vi "DriverStationSim_Comm_Loop.vi"(8 "error in (no error)":errorcluster) -> ()   [LabVIEW 2019, in "Trajectory_Library.lvlib"]
uses:
  Trajectory_Library.lvlib
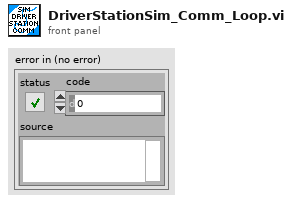
[diagram p1: front panel]
types:
  T1 = typedef "WPI_DriverStationRobotMode2.ctl" = enum16{"Autonomous Disabled", "Autonomous Enabled", "Teleop Disabled", "Teleop Enabled", "Disconnected", "Finish", "Test Disabled", "Test Enabled", "Emergency Stopped"}
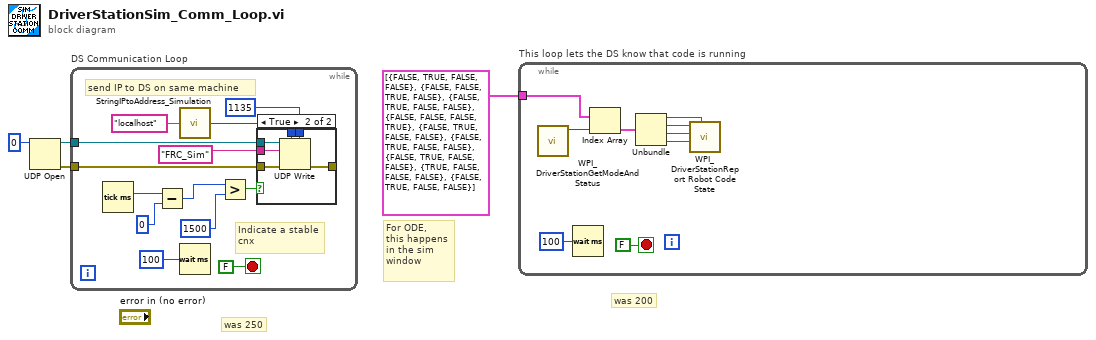
[diagram p0: block diagram]
diagram:
  # "was 200"
  # "was 250"
  # "For ODE,\nthis happens\nin the sim\nwindow"
  n1 = UDP Open(11:u16 0 ("port")) -> (port=w4:refnum<k16>, 0:w3:errorcluster)  [unwired: 4 in, 1 out]
  n2 = while "DS Communication Loop" {
    tunnel: w4 -> [w16]
    tunnel: w3 -> [w17]
    stop <- FALSE stop-if-true
    # "Indicate a stable\ncnx"
    # "send IP to DS on same machine"
    n3 = Tick Count (ms)() -> (millisecond timer value=w6:u32)
    n4 = Subtract(x=w6, y=u32 0) -> (x-y=w9:u32)
    n5 = call <vilib>:"StringIPtoAddress_Simulation.vi"("string IP"="localhost" ("DS IP 2")) -> ("address"=w13:u32)  [unwired: 14 in]
    n6 = Wait (ms)(milliseconds to wait=u32 100) -> ()  [unwired: 1 out]
    n7 = Greater?(x=w9, y=u32 1500 ("milliseconds to wait")) -> (0:w7:bool)
    n8 = case shown="True" w7 {
      tunnel: w17 -> [_ w23]
      tunnel: w16 -> [_ w22]
      tunnel: "FRC_Sim" ("data in") -> [_ w21]
      tunnel: w13 -> [_ w20]
      tunnel: [_ w19] -> _
      tunnel: u16 1135 ("port") -> [_ w18]
      frame False {
      }
      frame True {
        n9 = UDP Write(address=w20, port or service name=w18, connection ID=w22, data in=w21, 8:w23) -> (error out=w19:errorcluster)  [unwired: 1 in, 1 out]
      }
    }
  }
  n10 = while "This loop lets the DS know that code is running" {
    tunnel: cluster{bool, bool, bool, bool}[] [{FALSE, TRUE, FALSE, FALSE}, {FALSE, FALSE, TRUE, FALSE}, {FALSE, TRUE, FALSE, FALSE}, {FALSE, FALSE, FALSE, TRUE}, {FALSE, TRUE, FALSE, FALSE}, {FALSE, TRUE, FALSE, FALSE}, {FALSE, TRUE, FALSE, FALSE}, {TRUE, FALSE, FALSE, FALSE}, {FALSE, TRUE, FALSE, FALSE}] -> [w31]
    stop <- FALSE stop-if-true
    n11 = call <vilib>:"WPI_DriverStationGetModeAndStatus.vi"() -> ("Robot Mode"=w25:T1)  [unwired: 10 in, 1 out]
    n12 = Wait (ms)(milliseconds to wait=u32 100) -> ()  [unwired: 1 out]
    n13 = Index Array(array=w31, index=w25) -> (element=w26:cluster{bool, bool, bool, bool})
    n14 = Unbundle(w26) -> (w32:bool, w24:bool, w29:bool, w28:bool)
    n15 = call <vilib>:"WPI_DriverStationReport Robot Code State.vi"("Test"=w32, "TeleOp"=w28, "Autonomous"=w29, "Disabled"=w24) -> ()  [unwired: 7 in, 1 out]
  }
